vi "Get Config DOM Ref.vi"(8 "error in":errorcluster, 11 "System in":refnum<class "System.lvclass">) -> (0 "error out":errorcluster, 3 "System out":refnum<class "System.lvclass">)   [LabVIEW 2014, in "System.lvclass"]
uses:
  System.lvclass
  <vilib>/xml/Load XML File.vi
  <vilib>/xml/NI_XML.lvlib
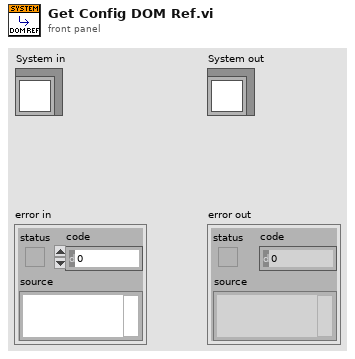
[diagram p1: front panel]
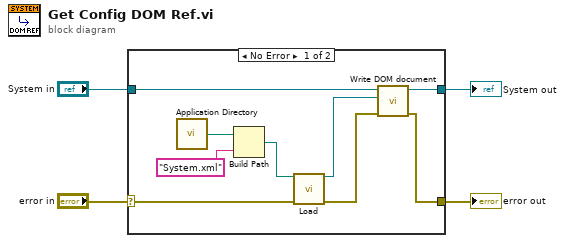
[diagram p0: block diagram]
diagram:
  n1 = case shown="No Error" "error in" {
    selector: "error in" -> [w9 w15]
    tunnel: [w5 w15] -> w3
    tunnel: [w8 w14] -> w1
    tunnel: "System in" -> [w13 w14]
    frame No Error {
      n2 = call <vilib>:"Application Directory.vi"() -> ("Application Directory"=w12:path)
      n3 = Build Path(base path=w12, name or relative path="System.xml") -> (appended path=w10:path)
      n4 = call-poly <vilib>:"Load.vi"("path to XML document"=w10, "error in (no error)"=w9) -> ("DOM document out"=w7:refnum<k20>, "error out"=w6:errorcluster)  [unwired: 11 in, 1 out]
      n5 = call-dynamic "Write DOM document.vi"("error in"=w6, "DOM document"=w7, "System in"=w13) -> ("error out"=w5:errorcluster, "System out"=w8:refnum<class "System.lvclass">)  [unwired: 7 in]
    }
    frame Error {
    }
  }
  "error out" <- w3
  "System out" <- w1
